vi "Do.vi"(8 "error in (no error)":errorcluster, 10 "Actor in":refnum<class "Actor.lvclass">, 11 "Configure Internal Trigger Rate [IT] Msg":refnum<class "Configure Internal Trigger Rate [IT] Msg.lvclass">) -> (0 "error out":errorcluster, 2 "Actor out":refnum<class "Actor.lvclass">)   [LabVIEW 2015, in "CS++Fgen.lvlib" / "Configure Internal Trigger Rate [IT] Msg.lvclass"]
doc: "This VI delivers the message to the actor by calling the appropriate method(s) on the actor."
uses:
  Configure Internal Trigger Rate [IT] Msg.lvclass
  <vilib>/ActorFramework/Actor/Actor.lvclass
  CS++Fgen/CS++Fgen.lvclass
  CSPP_Core/Actors/CS++PVMonitor Messages/CS++PVUpdate Msg/CS++PVUpdate Msg.lvclass/CS++PVUpdate Msg.ctl
  CSPP_Core/Classes/CS++ProcessVariables/ProcessVariable/PV.lvclass/PV.ctl
  Configure Internal Trigger Rate [IT] Msg.lvclass/Configure Internal Trigger Rate [IT] Msg.ctl
  CSPP_Core/Classes/CS++ProcessVariables/ProcessVariable/PV.lvclass
  CSPP_Core/Actors/CS++PVMonitor Messages/CS++PVUpdate Msg/CS++PVUpdate Msg.lvclass
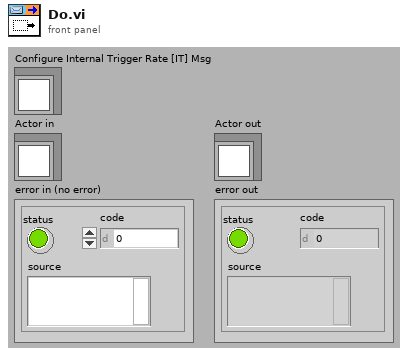
[diagram p1: front panel]
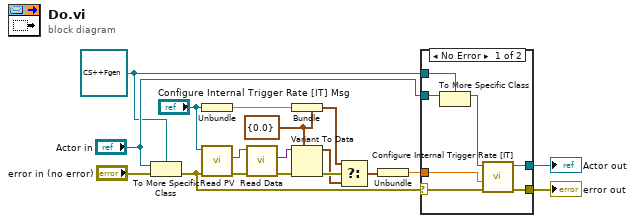
[diagram p0: block diagram]
diagram:
  w10 = cluster{"trigger rate (0.0 trig/sec)":dbl[unit]} {"trigger rate (0.0 trig/sec)"=0.0} ("Type")
  w14 = refnum<class "CS++Fgen.lvclass"> refnum ("Actor in")
  n1 = To More Specific Class(target class=w14, reference="Actor in", error in="error in (no error)") -> (error out=w3:errorcluster)  [unwired: 1 out]
  n2 = Unbundle ("Pre-Unbundler")("Configure Internal Trigger Rate [IT] Msg") -> (w1:dbl[unit])
  n3 = call "Read PV.vi"("error in (no error)"=w3, "CS++PVUpdate Msg in"="Configure Internal Trigger Rate [IT] Msg") -> ("error out"=w13:errorcluster, "PV"=w9:refnum<class "PV.lvclass">)  [unwired: 7 in, 1 out]
  n4 = call "Read Data.vi"("error in (no error)"=w13, "PV in"=w9) -> ("error out"=w7:errorcluster, "Data"=w8:variant)  [unwired: 7 in, 1 out]
  n5 = Bundle ("Pre-Bundler")(cluster=w10, "trigger rate (0.0 trig/sec)"=w1) -> (w11:cluster{"trigger rate (0.0 trig/sec)":dbl[unit]})
  n6 = Variant To Data(error in=w7, type=w10, Variant=w8) -> (data=w5:cluster{"trigger rate (0.0 trig/sec)":dbl[unit]}, error out=w12:errorcluster)
  n7 = Select ("MainSelect")(t=w11, s=w12, f=w5) -> (s? t:f=w6:cluster{"trigger rate (0.0 trig/sec)":dbl[unit]})
  n8 = Unbundle ("Main-Unbundler")(w6) -> ("trigger rate (0.0 trig/sec)"=w2:dbl[unit])
  n9 = case shown="No Error" w3 {
    selector: w3 -> [w23 w27]
    tunnel: [w25 w27] -> w17
    tunnel: [w24 w26] -> w16
    tunnel: "Actor in" -> [w22 w26]
    tunnel: w14 -> [w21 _]
    tunnel: w2 -> [w19 _]
    frame No Error {
      n10 = To More Specific Class(target class=w21, reference=w22) -> (specific class reference=w20:refnum<class "CS++Fgen.lvclass">)  [unwired: 1 in, 1 out]
      n11 = call "Configure Internal Trigger Rate [IT].vi"("error in (no error)"=w23, "trigger rate (0.0 trig/sec)"=w19, "CS++Fgen in"=w20) -> ("error out"=w25:errorcluster, "CS++Fgen out"=w24:refnum<class "CS++Fgen.lvclass">)  [unwired: 7 in]
    }
    frame Error {
    }
  }
  "error out" <- w17
  "Actor out" <- w16
